vi "Mem1024_Fast.vi"(8 "Init":bool, 9 "Phi2":bool, 10 "Phi1":bool, 11 "In":bool) -> (3 "Out":bool)   [LabVIEW 2012]
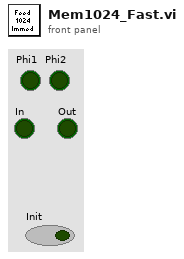
[diagram p1: front panel]
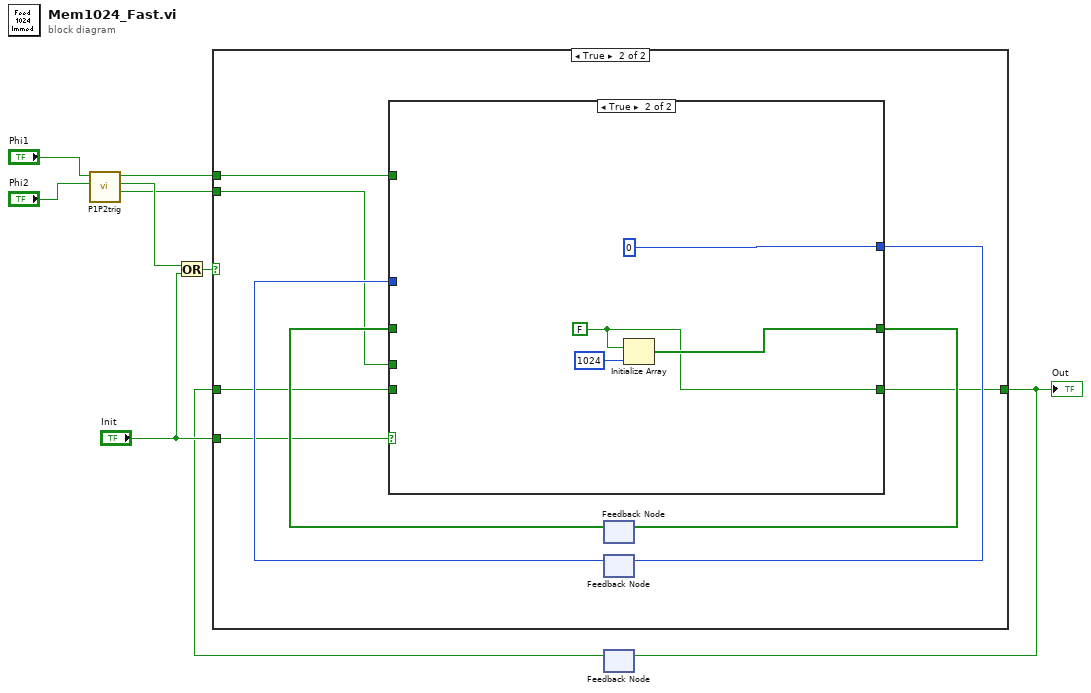
[diagram p0: block diagram]
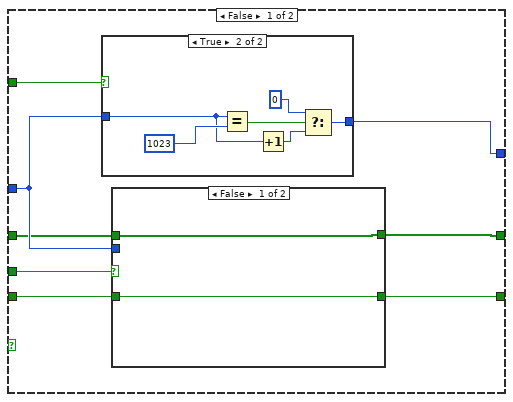
[diagram p3: hidden frame]
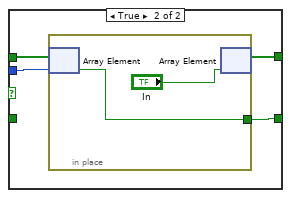
[diagram p4: hidden frame]
diagram:
  n1 = call "P1P2trig.vi"("Phi2"="Phi2", "Phi1"="Phi1") -> ("TrigUp"=w3:bool, "Clock"=w4:bool, "TrigDown"=w5:bool)  [unwired: 7 in]
  n2 = Or(x=w4, y="Init") -> (x .or. y?=w9:bool)
  n3 = feedback #1() -> (w1:bool)  [unwired: 1 in]
  n4 = case shown="True" w9 {
    tunnel: "Init" -> [_ w15]
    tunnel: w5 -> [_ w14]
    tunnel: w3 -> [_ w13]
    tunnel: [w10 w12] -> w2
    tunnel: w1 -> [w10 w11]
    frame False {
    }
    frame True {
      n5 = feedback #2() -> (w18:bool[])  [unwired: 1 in]
      n6 = feedback #3() -> (w16:i32)  [unwired: 1 in]
      n7 = case shown="True" w15 {
        tunnel: [w20 w45] -> w19
        tunnel: w18 -> [w21 _]
        tunnel: [w27 0] -> w17
        tunnel: w16 -> [w25 _]
        tunnel: [w23 w43] -> w12
        tunnel: w14 -> [w26 _]
        tunnel: w13 -> [w24 _]
        tunnel: w11 -> [w22 _]
        frame False {
          n8 = case shown="True" w26 {
            tunnel: w25 -> [w36 w37]
            tunnel: [w36 w39] -> w27
            frame False {
            }
            frame True {
              n9 = Equal?(x=w37, y=1023) -> (x = y?=w41:bool)
              n10 = Increment(x=w37) -> (x+1=w38:i32)
              n11 = Select(t=0 ("y"), s=w41, f=w38) -> (s? t:f=w39:i32)
            }
          }
          n12 = case shown="False" w24 {
            tunnel: w21 -> [w28 w33]
            tunnel: w25 -> [_ w32]
            tunnel: [w29 w31] -> w23
            tunnel: w22 -> [w29 _]
            tunnel: [w28 w30] -> w20
            frame False {
            }
            frame True {
              n13 = in-place {
                in-place-border: [w35] -> w31
                n14 = in-place-array #4(w33, w32) -> (w35:bool)
                n15 = in-place-array #4("In") -> (w30:bool[])  [unwired: 1 out]
              }
            }
          }
        }
        frame True {
          w43 = FALSE
          n16 = Initialize Array(w43, 1024 ("dimension size")) -> (w45:bool[])
        }
      }
      n17 = feedback-in #2(w19) -> ()
      n18 = feedback-in #3(w17) -> ()
    }
  }
  "Out" <- w2
  n19 = feedback-in #1(w2) -> ()
